vi "Tektronix_Model.vi"(0 "Oscilloscope-Change":bool=TRUE, 1 "TestIndex":i32, 2 "等待时间（毫秒）":u32, 3 "error in (no error)":errorcluster, 4 "Trigger Mode (0: Auto)":i32(ring) items=["Auto", "Normal"]) -> (5 "VISA resource name out":refnum<visa-resource-name>, 6 "error out":errorcluster)   [LabVIEW 2015]
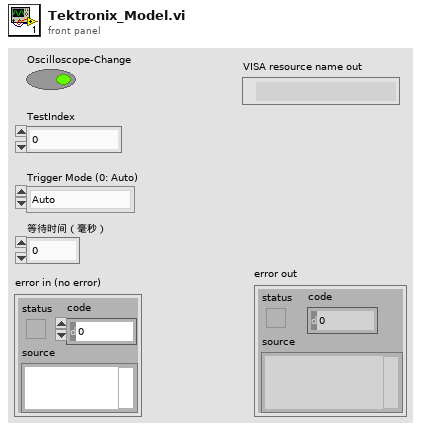
[diagram p1: front panel]
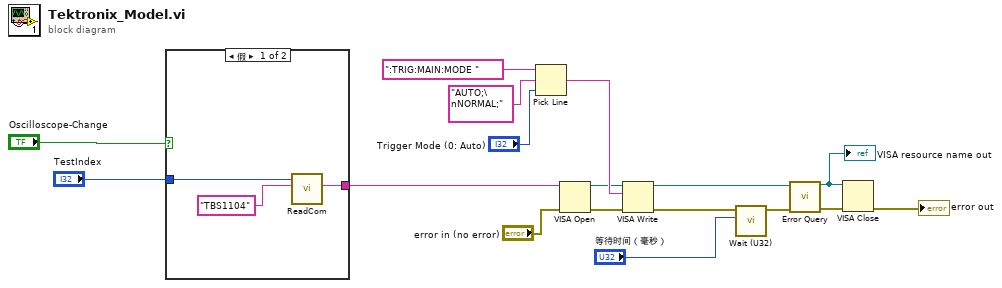
[diagram p0: block diagram]
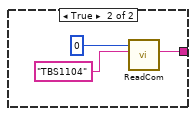
[diagram p2: hidden frame]
diagram:
  n1 = case shown="假" "Oscilloscope-Change" {
    tunnel: "TestIndex" -> [w18 _]
    tunnel: [w19 w21] -> w1
    frame False {
      n2 = call "ReadCom.vi"("仪器名称"="TBS1104", "MyIndex"=w18) -> ("COM"=w19:string)  [unwired: 7 in, 2 out]
    }
    frame True {
      n3 = call "ReadCom.vi"("仪器名称"="TBS1104", "MyIndex"=u8 0) -> ("COM"=w21:string)  [unwired: 7 in, 2 out]
    }
  }
  n4 = Pick Line(string ("")=":TRIG:MAIN:MODE ", multi-line string="AUTO;\nNORMAL;", line index="Trigger Mode (0: Auto)") -> (output string=w14:string)
  n5 = VISA Open(error in (no error)="error in (no error)", VISA resource name=w1) -> (VISA resource name=w9:refnum<visa-resource-name>, error out=w8:errorcluster)  [unwired: 3 in]
  n6 = VISA Write(VISA resource name=w9, write buffer=w14, error in (no error)=w8) -> (VISA resource name out=w17:refnum<visa-resource-name>, error out=w3:errorcluster)  [unwired: 1 out]
  n7 = call "Wait (U32).vi"("ms"="等待时间（毫秒）", "Error In"=w3) -> ("Error Out"=w4:errorcluster)  [unwired: 5 in]
  n8 = call "Error Query.vi"("error in (no error)"=w4, "VISA resource name"=w17) -> ("error out"=w12:errorcluster, "VISA resource name out"=w11:refnum<visa-resource-name>)  [unwired: 8 out]
  "VISA resource name out" <- w11
  n9 = VISA Close(VISA resource name=w11, error in (no error)=w12) -> (error out=→"error out":errorcluster)
